vi "log analysis_gps.vi"() -> ()   [LabVIEW 2018] (continued)
\t\n15:14:19.5\tlog_raw\tgps_raw\t\tsystem status\tnormal 2 28.100000 0 0\trobot status\t149.366560\t123.572297\t7.900100\t-1.132498\t-0.070564\t-2.751729\t0.265000\t0.072000\n\t\n15:14:20.0\tlog_raw\tgps_raw\t\tsystem status\tnormal 2 28.100000 0 0\trobot status\t149.509304\t123.554542\t7.903900\t-1.191642\t-0.071068\t-2.471488\t0.238000\t0.107000\n\t\n15:14:20.5\tlog_raw\tgps_raw\t\tsystem status\tnormal 2 28.100000 0 0\trobot status\t149.652416\t123.539883\t7.906600\t-1.338562\t-0.074577\t-2.215040\t0.346000\t-0.051000\n\t\n15:14:21.1\tlog_raw\tgps_raw\t\tsystem status\tnormal 2 28.100000 0 0\trobot status\t149.795480\t123.525074\t7.909900\t-1.415540\t-0.167405\t-1.900702\t0.334000\t-0.055000\n\t\n15:14:21.5\tlog_raw\tgps_raw\t\tsystem status\tnormal 2 28.100000 0 0\trobot status\t149.938796\t123.511245\t7.914500\t-1.445109\t-0.214035\t-1.639799\t0.448000\t-0.205000\n\t\n15:14:22.0\tlog_raw\tgps_raw\t\tsystem status\tnormal 2 28.100000 0 0\trobot status\t150.079264\t123.497692\t7.919300\t-1.431024\t-0.163741\t-1.401433\t0.206000\t0.151000\n\t\n15:14:22.6\tlog_raw\tgps_raw\t\tsystem status\tnormal 2 28.100000 0 0\trobot status\t150.220181\t123.485452\t7.922900\t-1.413802\t-0.077748\t-1.262179\t0.284000\t0.019000\n\t\n15:14:23.1\tlog_raw\tgps_raw\t\tsystem status\tnormal 2 28.100000 0 0\trobot status\t150.361255\t123.473733\t7.927200\t-1.413181\t-0.027253\t-1.156490\t0.330000\t-0.055000\n\t\n15:14:23.5\tlog_raw\tgps_raw\t\tsystem status\tnormal 2 28.100000 0 0\trobot status\t150.503771\t123.461894\t7.931500\t-1.372440\t0.029590\t-1.120872\t0.258000\t0.064000\n\t\n15:14:24.1\tlog_raw\tgps_raw\t\tsystem status\tnormal 2 28.200000 0 0\trobot status\t150.644323\t123.449417\t7.936600\t-1.282079\t0.146644\t-1.165071\t0.289000\t0.013000\n\t\n15:14:24.6\tlog_raw\tgps_raw\t\tsystem status\tnormal 2 28.200000 0 0\trobot status\t150.790773\t123.436712\t7.940900\t-1.280220\t0.083017\t-1.231244\t0.296000\t-0.010000\n\t\n15:14:25.1\tlog_raw\tgps_raw\t\tsystem status\tnormal 2 28.200000 0 0\trobot status\t150.935847\t123.423932\t7.945900\t-1.240454\t-0.005624\t-1.305863\t0.309000\t-0.012000\n\t\n15:14:25.6\tlog_raw\tgps_raw\t\tsystem status\tnormal 2 28.200000 0 0\trobot status\t151.077631\t123.412848\t7.950400\t-1.177343\t-0.073816\t-1.411200\t0.293000\t-0.008000\n\t\n15:14:26.1\tlog_raw\tgps_raw\t\tsystem status\tnormal 2 28.200000 0 0\trobot status\t151.222018\t123.401236\t7.955200\t-1.098789\t-0.167292\t-1.541033\t0.299000\t-0.021000\n\t\n15:14:26.6\tlog_raw\tgps_raw\t\tsystem status\tnormal 2 28.200000 0 0\trobot status\t151.363483\t123.388797\t7.959900\t-1.118551\t-0.220292\t-1.630374\t0.304000\t-0.009000\n\t\n15:14:27.1\tlog_raw\tgps_raw\t\tsystem status\tnormal 2 28.200000 0 0\trobot status\t151.503497\t123.375436\t7.964500\t-1.028524\t-0.208818\t-1.760086\t0.301000\t-0.013000\n\t\n15:14:27.6\tlog_raw\tgps_raw\t\tsystem status\tnormal 2 28.200000 0 0\trobot status\t151.642610\t123.361022\t7.970000\t-0.852113\t-0.242497\t-1.888728\t0.296000\t-0.013000\n\t\n15:14:28.1\tlog_raw\tgps_raw\t\tsystem status\tnormal 2 28.200000 0 0\trobot status\t151.788682\t123.345898\t7.975300\t-0.726687\t-0.323912\t-2.056816\t0.298000\t-0.019000\n\t\n15:14:28.6\tlog_raw\tgps_raw\t\tsystem status\tnormal 2 28.200000 0 0\trobot status\t151.931323\t123.331510\t7.978900\t-0.997430\t-0.231723\t-2.239434\t0.298000\t-0.017000\n\t\n15:14:29.1\tlog_raw\tgps_raw\t\tsystem status\tnormal 2 28.200000 0 0\trobot status\t152.077458\t123.315293\t7.983400\t-1.090482\t-0.103862\t-2.424222\t0.301000\t-0.020000\n\t\n15:14:29.6\tlog_raw\tgps_raw\t\tsystem status\tnormal 2 28.200000 0 0\trobot status\t152.221615\t123.296968\t7.987900\t-0.849760\t-0.011186\t-2.620059\t0.298000\t-0.016000\n\t\n15:14:30.1\tlog_raw\tgps_raw\t\tsystem status\tnormal 2 28.200000 0 0\trobot status\t152.368358\t123.277216\t7.992300\t-0.516595\t-0.224905\t-2.805522\t0.303000\t-0.008000\n\t\n15:14:30.6\tlog_raw\tgps_raw\t#INSPVAXA,USB3,0,48.5,FINESTEERING,2107,281688.600,02000000,471d,15824;INS_ALIGNMENT_COMPLETE,INS_RTKFIXED,37.37124079033,126.72255707314,7.9955,22.3000,-0.0400,0.2827,0.0199,-0.588574844,-0.376557071,93.100954007,0.4119,0.2777,0.5056,0.1103,0.0901,0.0751,0.1654,0.1662,5.1286,0f000001,0*54052947\n\tsystem status\tnormal 2 28.200000 0 0\trobot status\t152.529109\t123.257423\t7.995500\t-0.588575\t-0.376557\t-3.100954\t0.296000\t-0.006000\n\t\n15:14:31.1\tlog_raw\tgps_raw\t\tsystem status\tnormal 2 28.200000 0 0\trobot status\t152.659121\t123.241575\t7.999400\t-0.763688\t-0.674939\t-3.330027\t0.303000\t-0.016000\n\t\n15:14:31.6\tlog_raw\tgps_raw\t\tsystem status\tnormal 2 28.200000 0 0\trobot status\t152.805768\t123.221268\t8.003000\t-0.712582\t-0.950518\t-3.577154\t0.288000\t-0.020000\n\t\n15:14:32.1\tlog_raw\tgps_raw\t\tsystem status\tnormal 2 28.200000 0 0\trobot status\t152.951467\t123.200359\t8.007000\t-0.710267\t-0.843911\t-3.785734\t0.238000\t-0.109000\n\t\n15:14:32.6\tlog_raw\tgps_raw\t\tsystem status\tnormal 2 28.200000 0 0\trobot status\t153.091174\t123.178823\t8.009300\t-0.588136\t-0.683436\t-4.074866\t0.292000\t-0.015000\n\t\n15:14:33.1\tlog_raw\tgps_raw\t\tsystem status\tnormal 2 28.200000 0 0\trobot status\t153.233079\t123.156580\t8.011800\t-0.538851\t-0.581242\t-4.363275\t0.327000\t0.044000\n\t\n15:14:33.6\tlog_raw\tgps_raw\t\tsystem status\tnormal 2 28.200000 0 0\trobot status\t153.375195\t123.133242\t8.008900\t-0.412701\t-0.527172\t-4.622577\t0.360000\t0.118000\n\t\n15:14:34.1\tlog_raw\tgps_raw\t\tsystem status\tnormal 2 28.200000 0 0\trobot status\t153.517763\t123.109239\t8.007000\t-0.395813\t-0.605410\t-4.852309\t0.296000\t-0.002000\n\t\n15:14:34.6\tlog_raw\tgps_raw\t#INSPVAXA,USB3,0,49.0,FINESTEERING,2107,281692.600,02000000,471d,15824;INS_ALIGNMENT_COMPLETE,INS_RTKFIXED,37.37123920503,126.72256999557,8.0063,22.3000,-0.0578,0.2919,0.0133,-0.505898312,-0.718535643,95.167243727,0.4145,0.2869,0.5143,0.1104,0.0917,0.0756,0.1655,0.1660,5.1296,0f000001,0*c2aa46e2\n\tsystem status\tnormal 2 28.200000 0 0\trobot status\t153.673757\t123.081458\t8.006300\t-0.505898\t-0.718536\t-5.167244\t0.308000\t0.001000\n\t\n15:14:35.1\tlog_raw\tgps_raw\t\tsystem status\tnormal 2 28.200000 0 0\trobot status\t153.801573\t123.057376\t8.005800\t-0.487279\t-0.908052\t-5.339412\t0.294000\t-0.007000\n\t\n15:14:35.6\tlog_raw\tgps_raw\t\tsystem status\tnormal 2 28.200000 0 0\trobot status\t153.944107\t123.032631\t8.004700\t-0.547213\t-0.781307\t-5.501722\t0.296000\t0.001000\n\t\n15:14:36.1\tlog_raw\tgps_raw\t\tsystem status\tnormal 2 28.200000 0 0\trobot status\t154.084163\t123.006403\t8.003400\t-0.501860\t-0.671776\t-5.648809\t0.300000\t0.007000\n\t\n15:14:36.6\tlog_raw\tgps_raw\t\tsystem status\tnormal 2 28.200000 0 0\trobot status\t154.225777\t122.980167\t8.002400\t-0.527947\t-0.683883\t-5.812505\t0.302000\t0.006000\n\t\n15:14:37.1\tlog_raw\tgps_raw\t#INSPVAXA,USB3,0,47.0,FINESTEERING,2107,281695.100,02000000,471d,15824;INS_ALIGNMENT_COMPLETE,INS_RTKFIXED,37.37123802053,126.72257797318,8.0018,22.3000,-0.0593,0.2857,0.0050,-0.558480992,-0.544515597,95.936874114,0.4188,0.2924,0.5242,0.1107,0.0922,0.0760,0.1653,0.1660,5.1321,0f000001,0*63dd8461\n\tsystem status\tnormal 2 28.200000 0 0\trobot status\t154.380400\t122.949983\t8.001800\t-0.558481\t-0.544516\t-5.936874\t0.299000\t0.006000\n\t\n15:14:37.6\tlog_raw\tgps_raw\t\tsystem status\tnormal 2 28.200000 0 0\trobot status\t154.512542\t122.924219\t8.005400\t-0.525060\t-0.437586\t-6.058964\t0.298000\t0.015000\n\t\n15:14:38.1\tlog_raw\tgps_raw\t#INSPVAXA,USB3,0,50.0,FINESTEERING,2107,281696.100,02000000,471d,15824;INS_ALIGNMENT_COMPLETE,INS_RTKFIXED,37.37123750613,126.72258125435,8.0103,22.3000,-0.0675,0.2976,0.0099,-0.630143652,-0.426020851,96.136843189,0.4217,0.2975,0.5312,0.1110,0.0928,0.0763,0.1653,0.1661,5.1333,0f000001,0*1735351b\n\tsystem status\tnormal 2 28.200000 0 0\trobot status\t154.671041\t122.892888\t8.010300\t-0.630144\t-0.426021\t-6.136843\t0.308000\t0.011000\n\t\n15:14:38.6\tlog_raw\tgps_raw\t\tsystem status\tnormal 2 28.200000 0 0\trobot status\t154.810463\t122.866081\t8.012900\t-0.724588\t-0.515296\t-6.229481\t0.314000\t0.000000\n\t\n15:14:39.1\tlog_raw\tgps_raw\t#INSPVAXA,USB3,0,48.0,FINESTEERING,2107,281697.100,02000000,471d,15824;INS_ALIGNMENT_COMPLETE,INS_RTKFIXED,37.37123698193,126.72258460282,8.0164,22.3000,-0.0758,0.2921,0.0167,-0.785011326,-0.362402901,96.082518685,0.4231,0.3001,0.5368,0.1110,0.0930,0.0765,0.1653,0.1661,5.1347,0f000001,0*98f592bb\n\tsystem status\tnormal 2 28.100000 0 0\trobot status\t154.967643\t122.834704\t8.016400\t-0.785011\t-0.362403\t-6.082519\t0.300000\t0.016000\n\t\n15:14:39.6\tlog_raw\tgps_raw\t\tsystem status\tnormal 2 28.100000 0 0\trobot status\t155.092108\t122.811642\t8.019200\t-0.675963\t-0.233633\t-5.854448\t0.383000\t-0.117000\n\t\n15:14:40.1\tlog_raw\tgps_raw\t\tsystem status\tnormal 2 28.100000 0 0\trobot status\t155.232756\t122.785140\t8.022600\t-0.514960\t-0.265111\t-5.472110\t0.205000\t0.149000\n\t\n15:14:40.6\tlog_raw\tgps_raw\t#INSPVAXA,USB3,0,46.0,FINESTEERING,2107,281698.600,02000000,471d,15824;INS_ALIGNMENT_COMPLETE,INS_RTKFIXED,37.37123629785,126.72258936520,8.0229,22.3000,-0.0531,0.2999,0.0083,-0.429170205,-0.373001381,94.965510664,0.4234,0.2998,0.5394,0.1109,0.0928,0.0765,0.1652,0.1661,5.1363,0f000001,0*f47145af\n\tsystem status\tnormal 2 28.000000 0 0\trobot status\t155.389487\t122.758774\t8.022900\t-0.429170\t-0.373001\t-4.965511\t0.256000\t0.077000\n\t\n15:14:41.1\tlog_raw\tgps_raw\t#INSPVAXA,USB3,0,47.5,FINESTEERING,2107,281699.100,02000000,471d,15824;INS_ALIGNMENT_COMPLETE,INS_RTKFIXED,37.37123609876,126.72259093053,8.0227,22.3000,-0.0510,0.2765,0.0255,-0.446439369,-0.329194520,94.348853221,0.4489,0.3061,0.5623,0.1153,0.0940,0.0781,0.1653,0.1666,5.1379,0f000001,0*f0667120\n\tsystem status\tnormal 2 28.000000 0 0\trobot status\t155.528141\t122.736675\t8.022700\t-0.446439\t-0.329195\t-4.348853\t0.215000\t0.132000\n\t\n15:14:41.6\tlog_raw\tgps_raw\t#INSPVAXA,USB3,0,47.5,FINESTEERING,2107,281699.600,02000000,471d,15824;INS_ALIGNMENT_COMPLETE,INS_RTKFIXED,37.37123591668,126.72259250997,8.0220,22.3000,-0.0473,0.2889,0.0139,-0.571559626,-0.354554479,93.825556987,0.4489,0.3061,0.5623,0.1153,0.0940,0.0781,0.1653,0.1666,5.1379,0f000001,0*d2b474b3\n\tsystem status\tnormal 2 28.000000 0 0\trobot status\t155.668045\t122.716465\t8.022000\t-0.571560\t-0.354554\t-3.825557\t0.275000\t0.058000\n\t\n15:14:42.1\tlog_raw\tgps_raw\t\tsystem status\tnormal 2 28.000000 0 0\trobot status\t155.793898\t122.698945\t8.019900\t-0.596062\t-0.368937\t-3.271519\t0.265000\t0.070000\n\t\n15:14:42.6\tlog_raw\tgps_raw\t\tsystem status\tnormal 2 28.000000 0 0\trobot status\t155.937017\t122.681989\t8.015500\t-0.614799\t-0.508575\t-2.739622\t0.320000\t-0.011000\n\t\n15:14:43.1\tlog_raw\tgps_raw\t#INSPVAXA,USB3,0,46.5,FINESTEERING,2107,281701.100,02000000,471d,15824;INS_ALIGNMENT_COMPLETE,INS_RTKFIXED,37.37123543674,126.72259726700,8.0121,22.3000,-0.0545,0.2706,0.0002,-0.599049195,-0.261744490,92.339458537,0.4977,0.3169,0.6162,0.1213,0.0953,0.0812,0.1655,0.1673,5.1411,0f000001,0*bffa09db\n\tsystem status\tnormal 2 28.000000 0 0\trobot status\t156.089415\t122.663191\t8.012100\t-0.599049\t-0.261744\t-2.339459\t0.425000\t-0.170000\n\t\n15:14:43.6\tlog_raw\tgps_raw\t#INSPVAXA,USB3,0,46.5,FINESTEERING,2107,281701.600,02000000,471d,15824;INS_ALIGNMENT_COMPLETE,INS_RTKFIXED,37.37123527924,126.72259888049,8.0099,22.3000,-0.0672,0.2799,0.0012,-0.451214464,-0.240273754,91.937158376,0.4977,0.3169,0.6162,0.1213,0.0953,0.0812,0.1655,0.1673,5.1411,0f000001,0*07d7c6e7\n\tsystem status\tnormal 2 28.100000 0 0\trobot status\t156.232336\t122.645708\t8.009900\t-0.451214\t-0.240274\t-1.937158\t0.306000\t0.007000\n\t\n15:14:44.1\tlog_raw\tgps_raw\t#INSPVAXA,USB3,0,47.5,FINESTEERING,2107,281702.100,02000000,471d,15824;INS_ALIGNMENT_COMPLETE,INS_RTKFIXED,37.37123511620,126.72260050182,8.0076,22.3000,-0.0639,0.2800,0.0071,-0.195522404,-0.345413269,91.687324212,0.5177,0.3188,0.6402,0.1229,0.0952,0.0822,0.1654,0.1675,5.1426,0f000001,0*c86b297b\n\tsystem status\tnormal 2 28.100000 0 0\trobot status\t156.375950\t122.627610\t8.007600\t-0.195522\t-0.345413\t-1.687324\t0.323000\t-0.030000\n\t\n15:14:44.6\tlog_raw\tgps_raw\t#INSPVAXA,USB3,0,47.5,FINESTEERING,2107,281702.600,02000000,471d,15824;INS_ALIGNMENT_COMPLETE,INS_RTKFIXED,37.37123499980,126.72260210723,8.0027,22.3000,-0.0718,0.2769,0.0046,-0.302041493,-0.225202254,91.651416522,0.5177,0.3188,0.6402,0.1229,0.0952,0.0822,0.1654,0.1675,5.1426,0f000001,0*8e66a9f4\n\tsystem status\tnormal 2 28.100000 0 0\trobot status\t156.518155\t122.614689\t8.002700\t-0.302041\t-0.225202\t-1.651417\t0.357000\t-0.078000\n\t\n15:14:45.1\tlog_raw\tgps_raw\t#INSPVAXA,USB3,0,45.0,FINESTEERING,2107,281703.100,02000000,471d,15824;INS_ALIGNMENT_COMPLETE,INS_RTKFIXED,37.37123487466,126.72260370060,7.9985,22.3000,-0.0709,0.2986,0.0115,-0.451708680,-0.253518479,91.680936337,0.5338,0.3195,0.6613,0.1238,0.0951,0.0829,0.1654,0.1676,5.1442,0f000001,0*4cdf9694\n\tsystem status\tnormal 2 28.100000 0 0\trobot status\t156.659293\t122.600798\t7.998500\t-0.451709\t-0.253518\t-1.680936\t0.261000\t0.057000\n\t\n15:14:45.6\tlog_raw\tgps_raw\t#INSPVAXA,USB3,0,45.0,FINESTEERING,2107,281703.600,02000000,471d,15824;INS_ALIGNMENT_COMPLETE,INS_RTKFIXED,37.37123473881,126.72260531876,7.9953,22.3000,-0.0686,0.2839,0.0069,-0.545599376,-0.327030847,91.675911567,0.5338,0.3195,0.6613,0.1238,0.0951,0.0829,0.1654,0.1676,5.1442,0f000001,0*45031f18\n\tsystem status\tnormal 2 28.200000 0 0\trobot status\t156.802627\t122.585718\t7.995300\t-0.545599\t-0.327031\t-1.675912\t0.245000\t0.059000\n\t\n15:14:46.1\tlog_raw\tgps_raw\t#INSPVAXA,USB3,0,49.0,FINESTEERING,2107,281704.100,02000000,471d,15824;INS_ALIGNMENT_COMPLETE,INS_RTKFIXED,37.37123458474,126.72260693238,7.9920,22.3000,-0.0673,0.2665,0.0075,-0.425050811,-0.262256492,91.709435128,0.4707,0.3025,0.6068,0.1142,0.0929,0.0788,0.1651,0.1663,5.1457,0f000001,0*e320c835\n\tsystem status\tnormal 2 28.200000 0 0\trobot status\t156.945559\t122.568616\t7.992000\t-0.425051\t-0.262256\t-1.709435\t0.262000\t0.033000\n\t\n15:14:46.6\tlog_raw\tgps_raw\t#INSPVAXA,USB3,0,49.0,FINESTEERING,2107,281704.600,02000000,471d,15824;INS_ALIGNMENT_COMPLETE,INS_RTKFIXED,37.37123444909,126.72260850935,7.9897,22.3000,-0.0657,0.2780,0.0024,-0.316216564,-0.175738279,91.794051031,0.4707,0.3025,0.6068,0.1142,0.0929,0.0788,0.1651,0.1663,5.1457,0f000001,0*c024accc\n\tsystem status\tnormal 2 28.200000 0 0\trobot status\t157.085244\t122.553558\t7.989700\t-0.316217\t-0.175738\t-1.794051\t0.297000\t-0.006000\n\t\n15:14:47.1\tlog_raw\tgps_raw\t#INSPVAXA,USB3,0,48.5,FINESTEERING,2107,281705.100,02000000,471d,15824;INS_ALIGNMENT_COMPLETE,INS_RTKFIXED,37.37123430154,126.72261008444,7.9873,22.3000,-0.0633,0.2873,0.0036,-0.217542977,-0.113568421,91.893535267,0.4436,0.2955,0.5802,0.1116,0.0926,0.0771,0.1650,0.1661,5.1471,0f000001,0*d440002a\n\tsystem status\tnormal 2 28.200000 0 0\trobot status\t157.224763\t122.537180\t7.987300\t-0.217543\t-0.113568\t-1.893535\t0.298000\t-0.013000\n\t\n15:14:47.6\tlog_raw\tgps_raw\t#INSPVAXA,USB3,0,48.5,FINESTEERING,2107,281705.600,02000000,471d,15824;INS_ALIGNMENT_COMPLETE,INS_RTKFIXED,37.37123415162,126.72261168716,7.9829,22.3000,-0.0703,0.2649,-0.0005,-0.095589755,-0.218915380,92.040147564,0.4436,0.2955,0.5802,0.1116,0.0926,0.0771,0.1650,0.1661,5.1471,0f000001,0*3cc5b35f\n\tsystem status\tnormal 2 28.200000 0 0\trobot status\t157.366729\t122.520538\t7.982900\t-0.095590\t-0.218915\t-2.040148\t0.294000\t-0.018000\n\t\n15:14:48.1\tlog_raw\tgps_raw\t#INSPVAXA,USB3,0,47.0,FINESTEERING,2107,281706.100,02000000,471d,15824;INS_ALIGNMENT_COMPLETE,INS_RTKFIXED,37.37123399063,126.72261326131,7.9791,22.3000,-0.0689,0.2735,0.0004,-0.068217682,-0.338302495,92.198825064,0.4298,0.2917,0.5629,0.1111,0.0926,0.0763,0.1650,0.1662,5.1486,0f000001,0*0d2ba2e9\n\tsystem status\tnormal 2 28.200000 0 0\trobot status\t157.506165\t122.502668\t7.979100\t-0.068218\t-0.338302\t-2.198825\t0.297000\t-0.018000\n\t\n15:14:48.6\tlog_raw\tgps_raw\t#INSPVAXA,USB3,0,47.0,FINESTEERING,2107,281706.600,02000000,471d,15824;INS_ALIGNMENT_COMPLETE,INS_RTKFIXED,37.37123384411,126.72261483687,7.9751,22.3000,-0.0650,0.2968,0.0010,-0.179433418,-0.243858761,92.416884280,0.4298,0.2917,0.5629,0.1111,0.0926,0.0763,0.1650,0.1662,5.1486,0f000001,0*3a14ca69\n\tsystem status\tnormal 2 28.200000 0 0\trobot status\t157.645726\t122.486404\t7.975100\t-0.179433\t-0.243859\t-2.416884\t0.299000\t-0.016000\n\t\n15:14:49.1\tlog_raw\tgps_raw\t#INSPVAXA,USB3,0,46.5,FINESTEERING,2107,281707.100,02000000,471d,15824;INS_ALIGNMENT_COMPLETE,INS_RTKFIXED,37.37123367618,126.72261651459,7.9700,22.3000,-0.0663,0.2892,-0.0095,-0.200364886,-0.287717605,92.565518940,0.4222,0.2895,0.5502,0.1114,0.0926,0.0759,0.1650,0.1662,5.1501,0f000001,0*7d04a348\n\tsystem status\tnormal 2 28.200000 0 0\trobot status\t157.794335\t122.467764\t7.970000\t-0.200365\t-0.287718\t-2.565519\t0.296000\t-0.023000\n\t\n15:14:49.6\tlog_raw\tgps_raw\t#INSPVAXA,USB3,0,46.5,FINESTEERING,2107,281707.600,02000000,471d,15824;INS_ALIGNMENT_COMPLETE,INS_RTKFIXED,37.37123350681,126.72261819185,7.9654,22.3000,-0.0701,0.2829,0.0020,-0.131719254,-0.267188121,92.719108134,0.4222,0.2895,0.5502,0.1114,0.0926,0.0759,0.1650,0.1662,5.1501,0f000001,0*336f6954\n\tsystem status\tnormal 2 28.200000 0 0\trobot status\t157.942904\t122.448963\t7.965400\t-0.131719\t-0.267188\t-2.719108\t0.302000\t-0.017000\n\t\n15:14:50.1\tlog_raw\tgps_raw\t#INSPVAXA,USB3,0,46.5,FINESTEERING,2107,281708.100,02008000,471d,15824;INS_ALIGNMENT_COMPLETE,INS_RTKFIXED,37.37123332387,126.72261975086,7.9614,22.3000,-0.0675,0.2853,0.0025,-0.071583190,-0.126032206,92.932636241,0.4187,0.2881,0.5409,0.1120,0.0926,0.0757,0.1650,0.1662,5.1517,0f000001,0*717a5375\n\tsystem status\tnormal 2 28.200000 0 0\trobot status\t158.080999\t122.428657\t7.961400\t-0.071583\t-0.126032\t-2.932636\t0.304000\t-0.013000\n\t\n15:14:50.6\tlog_raw\tgps_raw\t#INSPVAXA,USB3,0,44.5,FINESTEERING,2107,281708.600,02008000,471d,15824;INS_ALIGNMENT_COMPLETE,INS_RTKFIXED,37.37123313227,126.72262135847,7.9570,22.3000,-0.0735,0.2879,0.0053,-0.006863606,-0.144876749,93.163596493,0.4187,0.2881,0.5409,0.1120,0.0926,0.0757,0.1650,0.1662,5.1517,0f000001,0*5328ad5b\n\tsystem status\tnormal 2 28.200000 0 0\trobot status\t158.223398\t122.407390\t7.957000\t-0.006864\t-0.144877\t-3.163596\t0.300000\t-0.019000\n\t\n15:14:51.1\tlog_raw\tgps_raw\t#INSPVAXA,USB3,0,45.0,FINESTEERING,2107,281709.100,02008000,471d,15824;INS_ALIGNMENT_COMPLETE,INS_RTKFIXED,37.37123292904,126.72262301314,7.9519,22.3000,-0.0859,0.2798,0.0008,-0.080624798,-0.243890207,93.431588866,0.4168,0.2866,0.5328,0.1122,0.0923,0.0756,0.1650,0.1661,5.1533,0f000001,0*5e6ee30b\n\tsystem status\tnormal 2 28.100000 0 0\trobot status\t158.369966\t122.384832\t7.951900\t-0.080625\t-0.243890\t-3.431589\t0.342000\t0.064000\n\t\n15:14:51.6\tlog_raw\tgps_raw\t#INSPVAXA,USB3,0,45.0,FINESTEERING,2107,281709.600,02008000,471d,15824;INS_ALIGNMENT_COMPLETE,INS_RTKFIXED,37.37123275225,126.72262461471,7.9473,22.3000,-0.0829,0.2713,-0.0040,-0.149358912,-0.219762797,93.778103830,0.4168,0.2866,0.5328,0.1122,0.0923,0.0756,0.1650,0.1661,5.1533,0f000001,0*a588a807\n\tsystem status\tnormal 2 28.100000 0 0\trobot status\t158.511831\t122.365208\t7.947300\t-0.149359\t-0.219763\t-3.778104\t0.296000\t-0.020000\n\t\n15:14:52.1\tlog_raw\tgps_raw\t#INSPVAXA,USB3,0,45.0,FINESTEERING,2107,281710.100,02008000,471d,15824;INS_ALIGNMENT_COMPLETE,INS_RTKFIXED,37.37123256909,126.72262620659,7.9441,22.3000,-0.0800,0.2841,-0.0050,-0.348638579,-0.216651585,94.159342839,0.4165,0.2852,0.5266,0.1124,0.0920,0.0756,0.1649,0.1660,5.1550,0f000001,0*bff3e08f\n\tsystem status\tnormal 2 28.100000 0 0\trobot status\t158.652837\t122.344877\t7.944100\t-0.348639\t-0.216652\t-4.159343\t0.305000\t-0.016000\n\t\n15:14:52.6\tlog_raw\tgps_raw\t#INSPVAXA,USB3,0,49.0,FINESTEERING,2107,281710.600,02008000,471d,15824;INS_ALIGNMENT_COMPLETE,INS_RTKFIXED,37.37123239058,126.72262777304,7.9409,22.3000,-0.0798,0.2944,-0.0023,-0.430611394,-0.234860716,94.547061846,0.4165,0.2852,0.5266,0.1124,0.0920,0.0756,0.1649,0.1660,5.1550,0f000001,0*d6308b3b\n\tsystem status\tnormal 2 28.100000 0 0\trobot status\t158.791590\t122.325063\t7.940900\t-0.430611\t-0.234861\t-4.547062\t0.252000\t-0.096000\n\t\n15:14:53.1\tlog_raw\tgps_raw\t#DUALANTENNAHEADINGA,USB3,0,48.0,FINESTEERING,2107,281711.100,02008000,d426,15824;SOL_COMPUTED,NARROW_FLOAT,-1.000000000,80.289344788,-44.356048584,0.0,300.718536377,180.000000000,\"631T\",19,8,8,8,04,00,20,23*d9de486e\n\tsystem status\tnormal 2 28.100000 0 0\trobot status\t158.929681\t122.303015\t7.937300\t-0.492200\t-0.313185\t-4.932154\t0.336000\t0.049000\n\t\n15:14:53.6\tlog_raw\tgps_raw\t#INSPVAXA,USB3,0,48.0,FINESTEERING,2107,281711.600,02008000,471d,15824;INS_ALIGNMENT_COMPLETE,INS_RTKFIXED,37.37123199532,126.72263088788,7.9365,22.3000,-0.0807,0.2590,-0.0074,-0.567150366,-0.272813348,95.297147623,0.4157,0.2838,0.5214,0.1122,0.0917,0.0756,0.1649,0.1659,5.1567,0f000001,0*5002614b\n\tsystem status\tnormal 2 28.100000 0 0\trobot status\t159.067498\t122.281190\t7.936500\t-0.567150\t-0.272813\t-5.297148\t0.277000\t-0.042000\n\t\n15:14:54.1\tlog_raw\tgps_raw\t#INSPVAXA,USB3,0,47.5,FINESTEERING,2107,281712.100,02000000,471d,15824;INS_ALIGNMENT_COMPLETE,INS_RTKFIXED,37.37123179004,126.72263242494,7.9368,22.3000,-0.0695,0.2725,-0.0019,-0.650599321,-0.130078123,95.641509239,0.4157,0.2825,0.5179,0.1119,0.0914,0.0757,0.1648,0.1658,5.1583,0f000001,0*44de4a90\n\tsystem status\tnormal 2 28.200000 0 0\trobot status\t159.203648\t122.258404\t7.936800\t-0.650599\t-0.130078\t-5.641509\t0.330000\t0.037000\n\t\n15:14:54.6\tlog_raw\tgps_raw\t#INSPVAXA,USB3,0,47.5,FINESTEERING,2107,281712.600,02000000,471d,15824;INS_ALIGNMENT_COMPLETE,INS_RTKFIXED,37.37123168411,126.72263304090,7.9346,22.3000,-0.0497,-0.0387,-0.0006,-0.768033993,-0.261504929,95.591408924,0.4157,0.2825,0.5179,0.1119,0.0914,0.0757,0.1648,0.1658,5.1583,0f000001,0*fe46b876\n\tsystem status\tnormal 2 28.200000 0 0\trobot status\t159.258209\t122.246647\t7.934600\t-0.768034\t-0.261505\t-5.591409\t0.000000\t0.000000\n\t\n15:14:55.1\tlog_raw\tgps_raw\t#INSPVAXA,USB3,0,49.0,FINESTEERING,2107,281713.100,02000000,471d,15824;INS_ALIGNMENT_COMPLETE,INS_RTKFIXED,37.37123162730,126.72263286916,7.9326,22.3000,-0.0467,-0.0089,-0.0011,-0.752184115,-0.247755356,95.681640614,0.4152,0.2811,0.5147,0.1145,0.0912,0.0757,0.1647,0.1656,5.1599,0f000001,0*7f213a14\n\tsystem status\tnormal 2 28.200000 0 0\trobot status\t159.242996\t122.240342\t7.932600\t-0.752184\t-0.247755\t-5.681641\t0.000000\t0.000000\n\t\n15:14:55.6\tlog_raw\tgps_raw\t#INSPVAXA,USB3,0,49.0,FINESTEERING,2107,281713.600,02000000,471d,15824;INS_ALIGNMENT_COMPLETE,INS_RTKFIXED,37.37123160226,126.72263284212,7.9312,22.3000,-0.0436,-0.0236,-0.0010,-0.754995173,-0.249841362,95.676005261,0.4152,0.2811,0.5147,0.1145,0.0912,0.0757,0.1647,0.1656,5.1599,0f000001,0*48133efc\n\tsystem status\tnormal 2 28.200000 0 0\trobot status\t159.240601\t122.237563\t7.931200\t-0.754995\t-0.249841\t-5.676005\t0.000000\t0.000000\n\t\n15:14:56.1\tlog_raw\tgps_raw\t#INSPVAXA,USB3,0,49.0,FINESTEERING,2107,281714.100,02000000,471d,15824;INS_ALIGNMENT_COMPLETE,INS_RTKFIXED,37.37123158399,126.72263279406,7.9298,22.3000,-0.0399,-0.0233,-0.0008,-0.760010437,-0.248532428,95.678009350,0.4172,0.2798,0.5120,0.1137,0.0910,0.0756,0.1647,0.1655,5.1584,0f000001,0*814e0d11\n\tsystem status\tnormal 2 28.200000 0 0\trobot status\t159.236344\t122.235535\t7.929800\t-0.760010\t-0.248532\t-5.678009\t0.000000\t0.000000\n\t\n15:14:56.6\tlog_raw\tgps_raw\t#INSPVAXA,USB3,0,49.0,FINESTEERING,2107,281714.600,02000000,471d,15824;INS_ALIGNMENT_COMPLETE,INS_RTKFIXED,37.37123160799,126.72263276180,7.9284,22.3000,-0.0364,-0.0240,-0.0004,-0.762178806,-0.247643160,95.688059791,0.4172,0.2798,0.5120,0.1137,0.0910,0.0756,0.1647,0.1655,5.1584,0f000001,0*b1bc14cf\n\tsystem status\tnormal 2 28.200000 0 0\trobot status\t159.233487\t122.238199\t7.928400\t-0.762179\t-0.247643\t-5.688060\t0.000000\t0.000000\n\t\n15:14:57.1\tlog_raw\tgps_raw\t#INSPVAXA,USB3,0,47.5,FINESTEERING,2107,281715.100,02000000,471d,15824;INS_ALIGNMENT_COMPLETE,INS_RTKFIXED,37.37123162975,126.72263271812,7.9272,22.3000,-0.0332,-0.0254,0.0000,-0.763298909,-0.246600758,95.701763966,0.4185,0.2789,0.5100,0.1127,0.0908,0.0756,0.1646,0.1655,5.1528,0f000001,0*0879a17d\n\tsystem status\tnormal 2 28.200000 0 0\trobot status\t159.229617\t122.240614\t7.927200\t-0.763299\t-0.246601\t-5.701764\t0.000000\t0.000000\n\t\n15:14:57.6\tlog_raw\tgps_raw\t#INSPVAXA,USB3,0,47.5,FINESTEERING,2107,281715.600,02000000,471d,15824;INS_ALIGNMENT_COMPLETE,INS_RTKFIXED,37.37123166929,126.72263269074,7.9254,22.3000,-0.0295,-0.0259,0.0000,-0.763181363,-0.245447561,95.720594560,0.4185,0.2789,0.5100,0.1127,0.0908,0.0756,0.1646,0.1655,5.1528,0f000001,0*8b144437\n\tsystem status\tnormal 2 28.200000 0 0\trobot status\t159.227192\t122.245003\t7.925400\t-0.763181\t-0.245448\t-5.720595\t0.000000\t0.000000\n\t\n15:14:58.1\tlog_raw\tgps_raw\t#INSPVAXA,USB3,0,47.5,FINESTEERING,2107,281716.100,02000000,471d,15824;INS_ALIGNMENT_COMPLETE,INS_RTKFIXED,37.37123170967,126.72263265292,7.9238,22.3000,-0.0264,-0.0269,-0.0004,-0.764362400,-0.245981262,95.737150322,0.4185,0.2781,0.5083,0.1118,0.0906,0.0755,0.1646,0.1654,5.1445,0f000001,0*f8e3de3b\n\tsystem status\tnormal 2 28.200000 0 0\trobot status\t159.223842\t122.249484\t7.923800\t-0.764362\t-0.245981\t-5.737150\t0.000000\t0.000000\n\t\n15:14:58.6\tlog_raw\tgps_raw\t#INSPVAXA,USB3,0,48.5,FINESTEERING,2107,281716.600,02000000,471d,15824;INS_ALIGNMENT_COMPLETE,INS_RTKFIXED,37.37123176851,126.72263264285,7.9224,22.3000,-0.0232,-0.0258,0.0004,-0.768584569,-0.246689742,95.757168230,0.4185,0.2781,0.5083,0.1118,0.0906,0.0755,0.1646,0.1654,5.1445,0f000001,0*4a6b11ff\n\tsystem status\tnormal 2 28.200000 0 0\trobot status\t159.222950\t122.256015\t7.922400\t-0.768585\t-0.246690\t-5.757168\t0.000000\t0.000000\n\t\n15:14:59.1\tlog_raw\tgps_raw\t#INSPVAXA,USB3,0,45.5,FINESTEERING,2107,281717.100,02000000,471d,15824;INS_ALIGNMENT_COMPLETE,INS_RTKFIXED,37.37123177555,126.72263328033,7.9223,22.3000,-0.0576,0.3644,0.0001,-0.832005766,-0.123893266,96.001595857,0.4179,0.2777,0.5069,0.1104,0.0904,0.0755,0.1645,0.1655,5.1359,0f000001,0*38e87445\n\tsystem status\tnormal 2 28.100000 0 0\trobot status\t159.279417\t122.256795\t7.922300\t-0.832006\t-0.123893\t-6.001596\t0.338000\t0.000000\n\t\n15:14:59.6\tlog_raw\tgps_raw\t#INSPVAXA,USB3,0,45.5,FINESTEERING,2107,281717.600,02000000,471d,15824;INS_ALIGNMENT_COMPLETE,INS_RTKFIXED,37.37123167276,126.72263519972,7.9226,22.3000,-0.0392,0.2146,0.0043,-0.709863436,-0.109995299,96.136679690,0.4179,0.2777,0.5069,0.1104,0.0904,0.0755,0.1645,0.1655,5.1359,0f000001,0*131293dc\n\tsystem status\tnormal 2 28.200000 0 0\trobot status\t159.449434\t122.245383\t7.922600\t-0.709863\t-0.109995\t-6.136680\t0.277000\t-0.009000\n\t\n15:15:00.1\tlog_raw\tgps_raw\t#INSPVAXA,USB3,0,50.0,FINESTEERING,2107,281718.100,02000000,471d,15824;INS_ALIGNMENT_COMPLETE,INS_RTKFIXED,37.37123162511,126.72263648434,7.9220,22.3000,-0.0555,0.3053,-0.0001,-0.719313500,0.029309323,96.356461624,0.4142,0.2776,0.5061,0.1102,0.0903,0.0754,0.1645,0.1655,5.1346,0f000001,0*65443b6e\n\tsystem status\tnormal 2 28.100000 0 0\trobot status\t159.563223\t122.240093\t7.922000\t-0.719314\t0.029309\t-6.356462\t0.317000\t-0.007000\n\t\n15:15:00.6\tlog_raw\tgps_raw\t#INSPVAXA,USB3,0,50.0,FINESTEERING,2107,281718.600,02000000,471d,15824;INS_ALIGNMENT_COMPLETE,INS_RTKFIXED,37.37123150821,126.72263819990,7.9208,22.3000,-0.0327,0.2368,0.0101,-0.836011591,-0.122473478,96.522319824,0.4142,0.2776,0.5061,0.1102,0.0903,0.0754,0.1645,0.1655,5.1346,0f000001,0*3c509359\n\tsystem status\tnormal 2 28.200000 0 0\trobot status\t159.715185\t122.227116\t7.920800\t-0.836012\t-0.122473\t-6.522320\t0.299000\t0.000000\n\t\n15:15:01.1\tlog_raw\tgps_raw\t#DUALANTENNAHEADINGA,USB3,0,50.0,FINESTEERING,2107,281719.100,02000000,d426,15824;SOL_COMPUTED,NARROW_FLOAT,-1.000000000,81.686454773,-57.139007568,0.0,241.198776245,172.427688599,\"631T\",19,9,9,9,04,00,20,23*98acc785\n\tsystem status\tnormal 2 28.200000 0 0\trobot status\t159.851512\t122.215460\t7.920300\t-0.991214\t-0.150939\t-6.766128\t0.309000\t-0.009000\n\t\n15:15:01.6\tlog_raw\tgps_raw\t#DUALANTENNAHEADINGA,USB3,0,50.5,FINESTEERING,2107,281719.600,02000000,d426,15824;SOL_COMPUTED,NARROW_FLOAT,-1.000000000,81.772033691,-56.640899658,0.0,242.991180420,178.717849731,\"631T\",19,9,9,9,04,00,20,23*247738d5\n\tsystem status\tnormal 2 28.200000 0 0\trobot status\t159.992006\t122.199768\t7.921100\t-1.016445\t-0.208647\t-6.964296\t0.295000\t-0.008000\n\t\n15:15:02.1\tlog_raw\tgps_raw\t#DUALANTENNAHEADINGA,USB3,0,50.5,FINESTEERING,2107,281720.100,02000000,d426,15824;SOL_COMPUTED,NARROW_FLOAT,-1.000000000,77.492141724,-53.828643799,0.0,241.831039429,180.000000000,\"631T\",18,8,8,8,04,00,20,23*d2631c09\n\tsystem status\tnormal 2 28.200000 0 0\trobot status\t160.139274\t122.180813\t7.921300\t-0.794888\t-0.384892\t-7.157644\t0.300000\t-0.015000\n\t\n15:15:02.6\tlog_raw\tgps_raw\t#INSPVAXA,USB3,0,50.5,FINESTEERING,2107,281720.600,02000000,471d,15824;INS_ALIGNMENT_COMPLETE,INS_RTKFIXED,37.37123091097,126.72264464380,7.9199,22.3000,-0.0398,0.2663,0.0043,-0.781491920,-0.508123165,97.323827994,0.4101,0.2774,0.5047,0.1107,0.0902,0.0753,0.1644,0.1655,5.1368,0f000001,0*f5b81503\n\tsystem status\tnormal 2 28.200000 0 0\trobot status\t160.285975\t122.160820\t7.919900\t-0.781492\t-0.508123\t-7.323828\t0.302000\t-0.017000\n\t\n15:15:03.1\tlog_raw\tgps_raw\t#INSPVAXA,USB3,0,44.0,FINESTEERING,2107,281721.100,02000000,471d,15824;INS_ALIGNMENT_COMPLETE,INS_RTKFIXED,37.37123072966,126.72264623422,7.9185,22.3000,-0.0371,0.2532,0.0002,-0.791450093,-0.646314917,97.497529339,0.4089,0.2773,0.5042,0.1108,0.0902,0.0752,0.1643,0.1654,5.1370,0f000001,0*861aa27e\n\tsystem status\tnormal 2 28.200000 0 0\trobot status\t160.426851\t122.140695\t7.918500\t-0.791450\t-0.646315\t-7.497529\t0.301000\t-0.009000\n\t\n15:15:03.6\tlog_raw\tgps_raw\t#INSPVAXA,USB3,0,44.0,FINESTEERING,2107,281721.600,02000000,471d,15824;INS_ALIGNMENT_COMPLETE,INS_RTKFIXED,37.37123052324,126.72264786246,7.9181,22.3000,-0.0351,0.2700,-0.0076,-0.812155960,-0.930405893,97.703567688,0.4089,0.2773,0.5042,0.1108,0.0902,0.0752,0.1643,0.1654,5.1370,0f000001,0*0ebef3fd\n\tsystem status\tnormal 2 28.200000 0 0\trobot status\t160.571078\t122.117783\t7.918100\t-0.812156\t-0.930406\t-7.703568\t0.301000\t-0.014000\n\t\n15:15:04.1\tlog_raw\tgps_raw\t#DUALANTENNAHEADINGA,USB3,0,44.0,FINESTEERING,2107,281722.100,02000000,d426,15824;SOL_COMPUTED,NARROW_FLOAT,-1.000000000,76.782913208,-57.608184814,0.0,174.641418457,168.358657837,\"631T\",20,9,9,9,04,00,20,23*2ea8cf0f\n\tsystem status\tnormal 2 28.200000 0 0\trobot status\t160.717291\t122.093027\t7.917000\t-0.823497\t-1.088152\t-7.893346\t0.304000\t-0.010000\n\t\n15:15:04.6\tlog_raw\tgps_raw\t#INSPVAXA,USB3,0,47.5,FINESTEERING,2107,281722.600,02000000,471d,15824;INS_ALIGNMENT_COMPLETE,INS_RTKFIXED,37.37123005820,126.72265110077,7.9161,22.3000,-0.0311,0.2570,0.0035,-0.906537656,-1.041249846,98.071868373,0.4085,0.2773,0.5040,0.1115,0.0902,0.0751,0.1642,0.1654,5.1358,0f000001,0*21f04e37\n\tsystem status\tnormal 2 28.200000 0 0\trobot status\t160.857922\t122.066165\t7.916100\t-0.906538\t-1.041250\t-8.071868\t0.298000\t-0.007000\n\t\n15:15:05.1\tlog_raw\tgps_raw\t#INSPVAXA,USB3,0,46.5,FINESTEERING,2107,281723.100,02000000,471d,15824;INS_ALIGNMENT_COMPLETE,INS_RTKFIXED,37.37122980766,126.72265265100,7.9163,22.3000,-0.0386,0.2513,-0.0019,-0.889198276,-0.870105161,98.274091102,0.4388,0.2808,0.5181,0.1159,0.0909,0.0762,0.1643,0.1660,5.1342,0f000001,0*96582036\n\tsystem status\tnormal 2 28.200000 0 0\trobot status\t160.995239\t122.038356\t7.916300\t-0.889198\t-0.870105\t-8.274091\t0.299000\t-0.007000\n\t\n15:15:05.6\tlog_raw\tgps_raw\t#INSPVAXA,USB3,0,46.5,FINESTEERING,2107,281723.600,02000000,471d,15824;INS_ALIGNMENT_COMPLETE,INS_RTKFIXED,37.37122953819,126.72265422237,7.9162,22.3000,-0.0387,0.2553,0.0003,-0.677469280,-0.596133835,98.468377537,0.4388,0.2808,0.5181,0.1159,0.0909,0.0762,0.1643,0.1660,5.1342,0f000001,0*0344c34f\n\tsystem status\tnormal 2 28.200000 0 0\trobot status\t161.134429\t122.008447\t7.916200\t-0.677469\t-0.596134\t-8.468378\t0.296000\t0.002000\n\t\n15:15:06.1\tlog_raw\tgps_raw\t#INSPVAXA,USB3,0,50.0,FINESTEERING,2107,281724.100,02000000,471d,15824;INS_ALIGNMENT_COMPLETE,INS_RTKFIXED,37.37122926408,126.72265582006,7.9155,22.3000,-0.0392,0.2664,0.0052,-0.552231420,-0.356374368,98.612981561,0.4681,0.2838,0.5347,0.1192,0.0914,0.0772,0.1643,0.1664,5.1316,0f000001,0*5ab7c900\n\tsystem status\tnormal 2 28.200000 0 0\trobot status\t161.275949\t121.978022\t7.915500\t-0.552231\t-0.356374\t-8.612982\t0.301000\t-0.002000\n\t\n15:15:06.6\tlog_raw\tgps_raw\t#DUALANTENNAHEADINGA,USB3,0,50.0,FINESTEERING,2107,281724.600,02000000,d426,15824;SOL_COMPUTED,NARROW_FLOAT,-1.000000000,73.725341797,-44.577819824,0.0,216.156219482,180.000000000,\"631T\",18,6,6,6,04,00,20,03*eb9ec7a2\n\tsystem status\tnormal 2 28.200000 0 0\trobot status\t161.408583\t121.948574\t7.916500\t-0.654606\t-0.102686\t-8.784986\t0.295000\t0.011000\n\t\n15:15:07.1\tlog_raw\tgps_raw\t#DUALANTENNAHEADINGA,USB3,0,48.0,FINESTEERING,2107,281725.100,02000000,d426,15824;SOL_COMPUTED,NARROW_FLOAT,-1.000000000,77.386466980,-38.596252441,0.0,347.977569580,180.000000000,\"631T\",17,7,7,6,04,00,20,33*9a5ac747\n\tsystem status\tnormal 2 28.200000 0 0\trobot status\t161.543202\t121.918259\t7.919400\t-0.700530\t0.057698\t-8.915070\t0.298000\t0.003000\n\t\n15:15:07.6\tlog_raw\tgps_raw\t#DUALANTENNAHEADINGA,USB3,0,48.0,FINESTEERING,2107,281725.600,02000000,d426,15824;SOL_COMPUTED,NARROW_FLOAT,-1.000000000,74.226867676,-38.265563965,0.0,314.182830811,180.000000000,\"631T\",17,7,7,6,04,00,20,23*45cb672d\n\tsystem status\tnormal 2 28.200000 0 0\trobot status\t161.685620\t121.886779\t7.924500\t-0.616560\t-0.013012\t-8.952659\t0.298000\t0.008000\n\t\n15:15:08.1\tlog_raw\tgps_raw\t#DUALANTENNAHEADINGA,USB3,0,48.0,FINESTEERING,2107,281726.100,02000000,d426,15824;SOL_COMPUTED,NARROW_FLOAT,-1.000000000,204.498168945,55.872886658,0.0,207.629287720,89.946952820,\"631T\",18,5,5,5,04,00,20,03*b03bb7fc\n\tsystem status\tnormal 2 28.200000 0 0\trobot status\t161.789883\t121.860793\t7.929500\t-0.487258\t-0.169488\t-9.052750\t0.000000\t0.000000\n\t\n15:15:08.6\tlog_raw\tgps_raw\t#DUALANTENNAHEADINGA,USB3,0,49.5,FINESTEERING,2107,281726.600,02000000,d426,15824;SOL_COMPUTED,NARROW_FLOAT,-1.000000000,205.496963501,57.094558716,0.0,186.765380859,78.783508301,\"631T\",22,5,5,5,04,00,20,03*8aea4973\n\tsystem status\tnormal 2 28.200000 0 0\trobot status\t161.746265\t121.859693\t7.931300\t-0.554375\t0.015983\t-8.987698\t-0.008000\t-0.012000\n\t\n15:15:09.1\tlog_raw\tgps_raw\t#INSPVAXA,USB3,0,40.0,FINESTEERING,2107,281727.100,02000000,471d,15824;INS_ALIGNMENT_COMPLETE,INS_RTKFIXED,37.37122812563,126.72266113643,7.9335,22.3000,-0.0046,-0.0366,0.0030,-0.538484803,-0.008426097,98.999278684,0.4214,0.2780,0.5150,0.1122,0.0902,0.0752,0.1639,0.1653,5.1250,0f000001,0*ffbd65c8\n\tsystem status\tnormal 2 28.200000 0 0\trobot status\t161.746865\t121.851662\t7.933500\t-0.538485\t-0.008426\t-8.999279\t-0.002000\t-0.003000\n\t\n15:15:09.6\tlog_raw\tgps_raw\t#DUALANTENNAHEADINGA,USB3,0,40.0,FINESTEERING,2107,281727.600,02000000,d426,15824;SOL_COMPUTED,NARROW_FLOAT,-1.000000000,200.788482666,48.749797821,0.0,300.075164795,180.000000000,\"631T\",21,7,7,7,04,00,20,33*2f30a934\n\tsystem status\tnormal 2 28.200000 0 0\trobot status\t161.746437\t121.846603\t7.934500\t-0.539060\t-0.010265\t-8.999947\t0.000000\t0.000000\n\t\n15:15:10.1\tlog_raw\tgps_raw\t#DUALANTENNAHEADINGA,USB3,0,40.0,FINESTEERING,2107,281728.100,02000000,d426,15824;SOL_COMPUTED,NARROW_FLOAT,-1.000000000,68.682434082,-18.649810791,0.0,214.877609253,180.000000000,\"631T\",24,9,9,7,04,00,20,33*477f08c5\n\tsystem status\tnormal 2 28.200000 0 0\trobot status\t161.745769\t121.842520\t7.935000\t-0.538763\t-0.010484\t-9.003599\t0.000000\t0.000000\n\t\n15:15:10.6\tlog_raw\tgps_raw\t#INSPVAXA,USB3,0,47.5,FINESTEERING,2107,281728.600,02000000,471d,15824;INS_ALIGNMENT_COMPLETE,INS_RTKFIXED,37.37122802316,126.72266112148,7.9338,22.3000,-0.0028,-0.0273,0.0028,-0.537660493,-0.013430681,99.001211572,0.4185,0.2775,0.5119,0.1116,0.0903,0.0750,0.1638,0.1653,5.1258,0f000001,0*537c1130\n\tsystem status\tnormal 2 28.200000 0 0\trobot status\t161.745541\t121.840290\t7.933800\t-0.537660\t-0.013431\t-9.001212\t0.000000\t0.000000\n\t\n15:15:11.1\tlog_raw\tgps_raw\t#DUALANTENNAHEADINGA,USB3,0,40.0,FINESTEERING,2107,281729.100,02000000,d426,15824;SOL_COMPUTED,NARROW_FLOAT,-1.000000000,109.638298035,-31.887359619,0.0,360.000000000,180.000000000,\"631T\",23,10,10,8,04,00,20,33*61c9d85b\n\tsystem status\tnormal 2 28.200000 0 0\trobot status\t161.744418\t121.838806\t7.932500\t-0.538592\t-0.014051\t-9.002299\t0.000000\t0.000000\n\t\n15:15:11.6\tlog_raw\tgps_raw\t#DUALANTENNAHEADINGA,USB3,0,40.0,FINESTEERING,2107,281729.600,02000000,d426,15824;SOL_COMPUTED,NARROW_FLOAT,-1.000000000,110.155059814,-31.497802734,0.0,360.000000000,180.000000000,\"631T\",22,10,10,8,04,00,20,23*86070080\n\tsystem status\tnormal 2 28.200000 0 0\trobot status\t161.744784\t121.839135\t7.931100\t-0.538261\t-0.015804\t-9.004777\t0.000000\t0.000000\n\t\n15:15:12.1\tlog_raw\tgps_raw\t#DUALANTENNAHEADINGA,USB3,0,40.0,FINESTEERING,2107,281730.100,02000000,d426,15824;SOL_COMPUTED,NARROW_FLOAT,-1.000000000,72.987403870,-66.832275391,0.0,145.125228882,72.779129028,\"631T\",22,9,9,9,04,00,20,33*22d7f0e2\n\tsystem status\tnormal 2 28.200000 0 0\trobot status\t161.744277\t121.840253\t7.930000\t-0.538223\t-0.015972\t-9.008248\t0.000000\t0.000000\n\t\n15:15:12.6\tlog_raw\tgps_raw\t#DUALANTENNAHEADINGA,USB3,0,44.5,FINESTEERING,2107,281730.600,02000000,d426,15824;SOL_COMPUTED,NARROW_FLOAT,-1.000000000,73.134811401,-67.340759277,0.0,145.030975342,70.451110840,\"631T\",24,8,8,8,04,00,20,23*a3bb5097\n\tsystem status\tnormal 2 28.200000 0 0\trobot status\t161.745905\t121.842579\t7.929100\t-0.537707\t-0.018375\t-9.012536\t0.000000\t0.000000\n\t\n15:15:13.1\tlog_raw\tgps_raw\t#DUALANTENNAHEADINGA,USB3,0,44.5,FINESTEERING,2107,281731.100,02000000,d426,15824;SOL_COMPUTED,NARROW_FLOAT,-1.000000000,67.550712585,-53.724426270,0.0,93.597503662,81.789405823,\"631T\",24,11,11,8,04,00,20,33*f2cdb2de\n\tsystem status\tnormal 2 28.200000 0 0\trobot status\t161.746893\t121.845330\t7.928100\t-0.537452\t-0.016854\t-9.014789\t0.000000\t0.000000\n\t\n15:15:13.6\tlog_raw\tgps_raw\t#DUALANTENNAHEADINGA,USB3,0,46.0,FINESTEERING,2107,281731.600,02000000,d426,15824;SOL_COMPUTED,NARROW_FLOAT,-1.000000000,67.703987122,-53.717529297,0.0,93.903839111,81.812553406,\"631T\",25,11,11,8,04,00,20,33*84af30bc\n\tsystem status\tnormal 2 28.200000 0 0\trobot status\t161.748678\t121.847835\t7.926700\t-0.537067\t-0.017297\t-9.017826\t0.002000\t0.003000\n\t\n15:15:14.1\tlog_raw\tgps_raw\t#DUALANTENNAHEADINGA,USB3,0,46.0,FINESTEERING,2107,281732.100,02000000,d426,15824;SOL_COMPUTED,NARROW_FLOAT,-1.000000000,70.648727417,-51.742156982,0.0,100.178024292,90.939315796,\"631T\",24,9,9,8,04,00,20,33*a1cde6a3\n\tsystem status\tnormal 2 28.100000 0 0\trobot status\t161.848152\t121.835574\t7.927700\t-0.619627\t0.169508\t-8.962036\t0.333000\t0.037000\n\t\n15:15:14.6\tlog_raw\tgps_raw\t#DUALANTENNAHEADINGA,USB3,0,48.5,FINESTEERING,2107,281732.600,02000000,d426,15824;SOL_COMPUTED,NARROW_FLOAT,-1.000000000,71.467155457,-52.314849854,0.0,103.026306152,90.018371582,\"631T\",24,9,9,7,04,00,20,33*b7826648\n\tsystem status\tnormal 2 28.200000 0 0\trobot status\t161.999751\t121.813811\t7.928200\t-0.700768\t0.278769\t-8.977023\t0.281000\t-0.020000\n\t\n15:15:15.1\tlog_raw\tgps_raw\t#DUALANTENNAHEADINGA,USB3,0,46.5,FINESTEERING,2107,281733.100,02000000,d426,15824;SOL_COMPUTED,NARROW_FLOAT,-1.000000000,126.205139160,18.349567413,0.0,360.000000000,180.000000000,\"631T\",24,8,8,7,04,00,20,33*2d8a4dce\n\tsystem status\tnormal 2 28.100000 0 0\trobot status\t162.146267\t121.792105\t7.930200\t-0.610006\t0.302068\t-8.737765\t0.311000\t-0.012000\n\t\n15:15:15.6\tlog_raw\tgps_raw\t#DUALANTENNAHEADINGA,USB3,0,46.5,FINESTEERING,2107,281733.600,
